vi "ep_Initialize Parameters.vi"(4 "current#":i32, 5 "harmonic order to calibrate":u32[](array[numeric]), 6 "voltage#":i32, 7 "frequency [Hz]":dbl=50.0 format="%_6g", 8 "ranges to calibrate spectra [%]":dbl[](array[numeric]), 9 "ranges to calibrate gains [%]":dbl[](array[numeric]), 10 "current full-range RMS value":dbl=5.0, 11 "voltage full-range RMS value":dbl=300.0) -> (3 "calibration parameters":T1)   [LabVIEW 2012]
uses:
  <vilib>/addons/Electrical Power/Example Support/PQ/Calibration/ep_Calibration.ctl
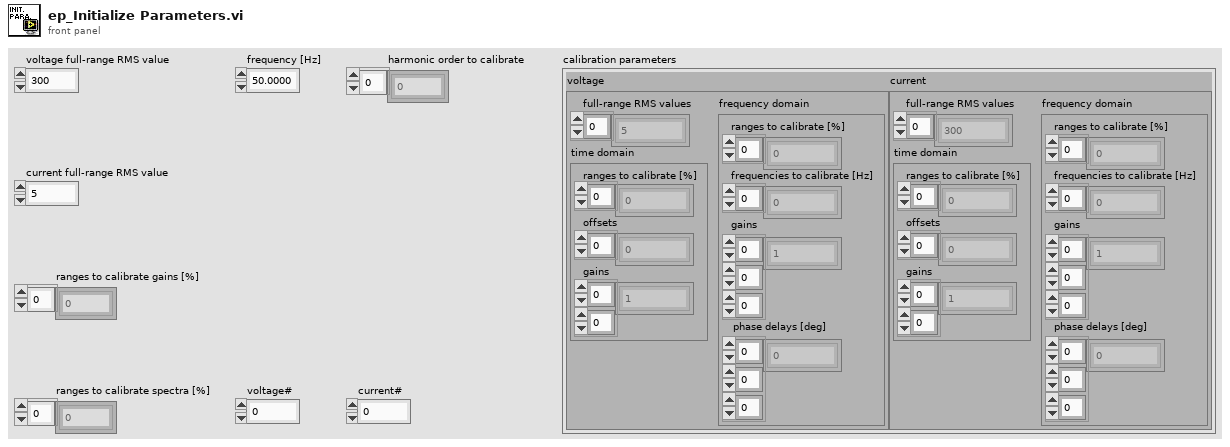
[diagram p1: front panel]
types:
  T1 = typedef "ep_Calibration.ctl" = cluster{"voltage":cluster{"full-range RMS values":dbl[], "time domain":cluster{"ranges to calibrate [%]":dbl[], "offsets":dbl[], "gains":dbl[][]}, "frequency domain":cluster{"ranges to calibrate [%]":dbl[], "frequencies to calibrate [Hz]":dbl[], "phase delays [deg]":dbl[][][], "gains":dbl[][][]}}, "current":cluster{"full-range RMS values":dbl[], "time domain":cluster{"ranges to calibrate [%]":dbl[], "offsets":dbl[], "gains":dbl[][]}, "frequency domain":cluster{"ranges to calibrate [%]":dbl[], "frequencies to calibrate [Hz]":dbl[], "phase delays [deg]":dbl[][][], "gains":dbl[][][]}}}
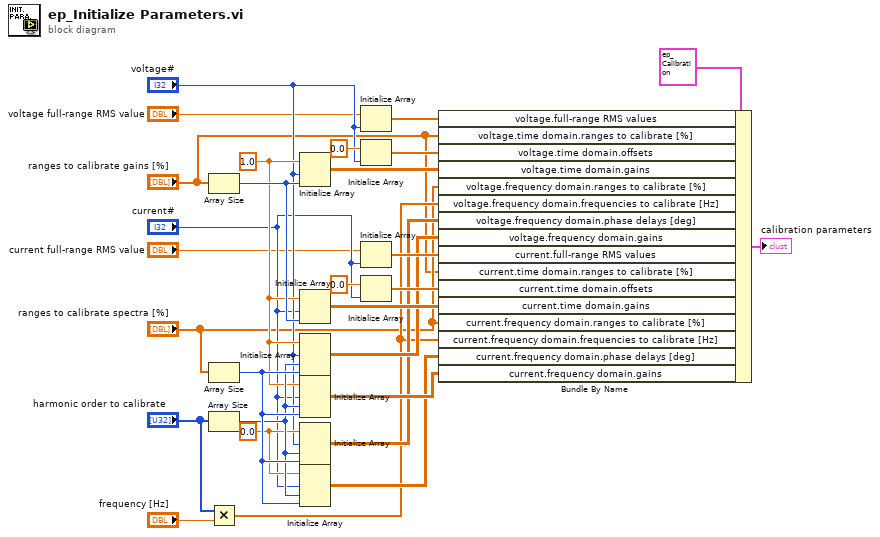
[diagram p0: block diagram]
diagram:
  w16 = 0.0
  w10 = 1.0
  n1 = Array Size(array="ranges to calibrate gains [%]") -> (size(s)=w25:i32)
  n2 = Array Size(array="ranges to calibrate spectra [%]") -> (size(s)=w18:i32)
  n3 = Array Size(array="harmonic order to calibrate") -> (size(s)=w17:i32)
  n4 = Multiply(x="harmonic order to calibrate", y="frequency [Hz]") -> (x*y=w11:dbl[])
  n5 = Initialize Array(w10, "voltage#", w25) -> (w24:dbl[][])
  n6 = Initialize Array(w10, "current#", w25) -> (w23:dbl[][])
  n7 = Initialize Array(w10, "voltage#", w17, w18) -> (w15:dbl[][][])
  n8 = Initialize Array(w10, "current#", w17, w18) -> (w14:dbl[][][])
  n9 = Initialize Array(w16, "voltage#", w17, w18) -> (w13:dbl[][][])
  n10 = Initialize Array(w16, "current#", w17, w18) -> (w12:dbl[][][])
  n11 = Initialize Array("voltage full-range RMS value", "voltage#") -> (w27:dbl[])
  n12 = Initialize Array(0.0 ("element"), "voltage#") -> (w22:dbl[])
  n13 = Initialize Array("current full-range RMS value", "current#") -> (w26:dbl[])
  n14 = Initialize Array(0.0 ("element"), "current#") -> (w20:dbl[])
  n15 = Bundle By Name(cluster=T1 {"voltage"={"full-range RMS values"=[], "time domain"={"ranges to calibrate [%]"=[], "offsets"=[], "gains"=[]}, "frequency domain"={"ranges to calibrate [%]"=[], "frequencies to calibrate [Hz]"=[], "phase delays [deg]"=[], "gains"=[]}}, "current"={"full-range RMS values"=[], "time domain"={"ranges to calibrate [%]"=[], "offsets"=[], "gains"=[]}, "frequency domain"={"ranges to calibrate [%]"=[], "frequencies to calibrate [Hz]"=[], "phase delays [deg]"=[], "gains"=[]}}} ("Clear"), "voltage.full-range RMS values"=w27, "voltage.time domain.ranges to calibrate [%]"="ranges to calibrate gains [%]", "voltage.time domain.offsets"=w22, "voltage.time domain.gains"=w24, "voltage.frequency domain.ranges to calibrate [%]"="ranges to calibrate spectra [%]", "voltage.frequency domain.frequencies to calibrate [Hz]"=w11, "voltage.frequency domain.phase delays [deg]"=w13, "voltage.frequency domain.gains"=w15, "current.full-range RMS values"=w26, "current.time domain.ranges to calibrate [%]"="ranges to calibrate gains [%]", "current.time domain.offsets"=w20, "current.time domain.gains"=w23, "current.frequency domain.ranges to calibrate [%]"="ranges to calibrate spectra [%]", "current.frequency domain.frequencies to calibrate [Hz]"=w11, "current.frequency domain.phase delays [deg]"=w12, "current.frequency domain.gains"=w14) -> (→"calibration parameters":T1)
